vi "Array2HSVColorPic.vi"(0 "Intensity":dbl[][](array[numeric]), 1 "Threshold (max)":dbl, 2 "Threshold (min)":dbl, 3 "Lifetime":dbl[][](array[numeric]), 4 "lifetime_max (s)":dbl=1e-05, 5 "lifetime_min (s)":dbl, 6 "Pic Reference":refnum<vi>, 7 "Auto Scale?":bool) -> (14 "Gray Picture":picture caption="HSV to RGB Picture")   [LabVIEW 2018]
uses:
  <vilib>/picture/picture.llb/Draw True-Color Pixmap.vi
panel:
  in  "hue_min [red]":dbl
  in  "hue_max [blue]":dbl=0.7
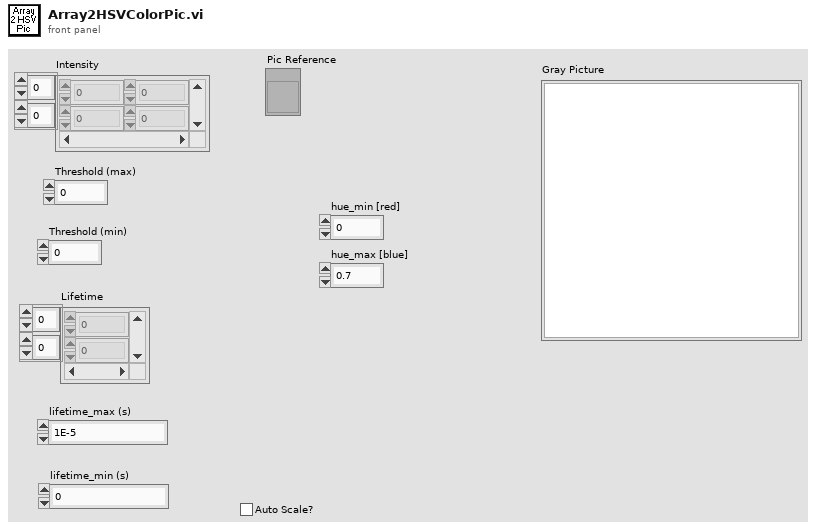
[diagram p1: front panel]
types:
  T1 = typedef "LVBoundsTypeDef.ctl" = cluster{"Width":u32, "Height":u32}
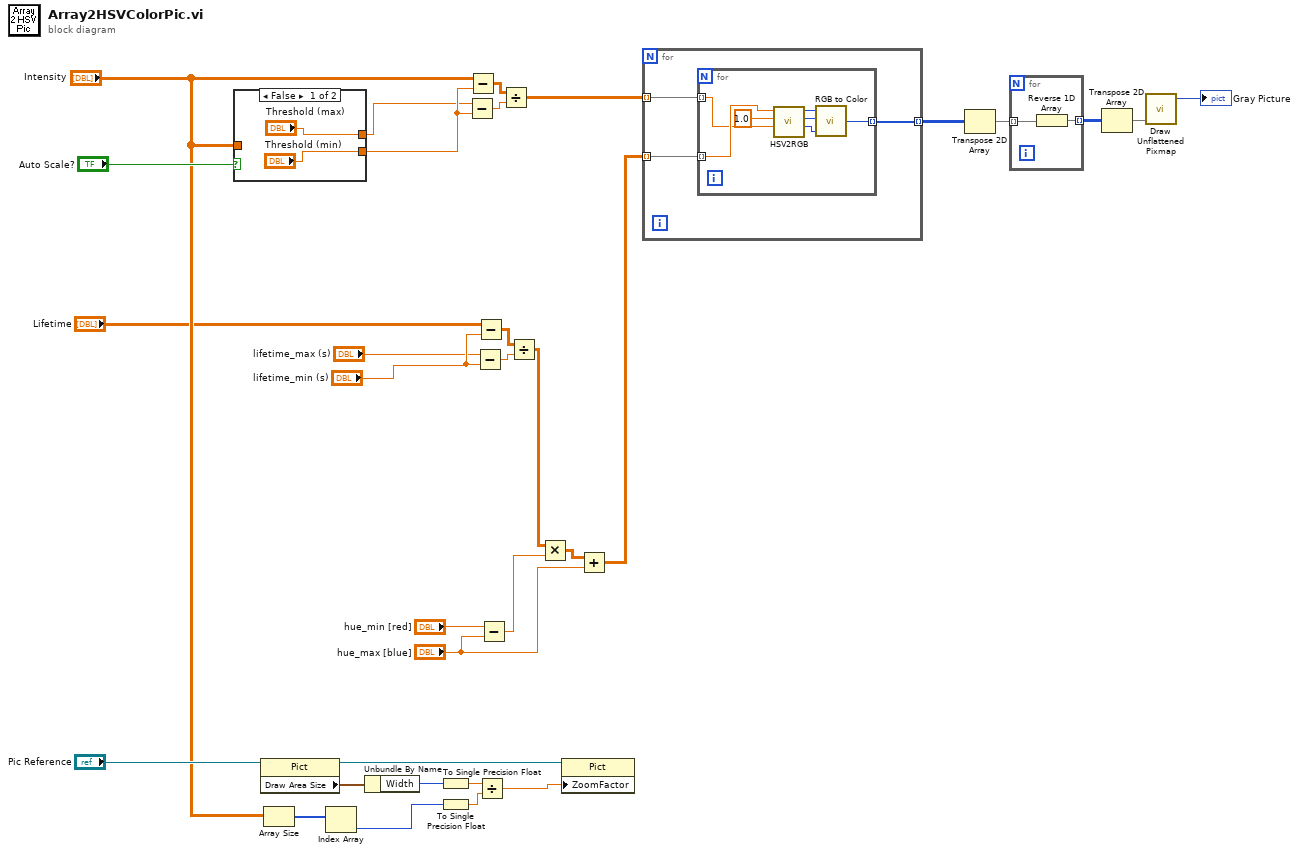
[diagram p0: block diagram]
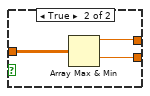
[diagram p2: hidden frame]
diagram:
  n1 = case shown="False" "Auto Scale?" {
    tunnel: "Intensity" -> [_ w37]
    tunnel: ["Threshold (max)" w36] -> w28
    tunnel: ["Threshold (min)" w35] -> w29
    frame False {
    }
    frame True {
      n2 = Array Max & Min(array=w37) -> (max value=w36:dbl, min value=w35:dbl)  [unwired: 2 out]
    }
  }
  n3 = property on="Property Node" class="Pict"(reference="Pic Reference") -> (reference out=w17:refnum<vi>, "Draw Area Size"=w19:T1)  [unwired: 1 in, 1 out]
  n4 = Array Size(array="Intensity") -> (size(s)=w15:i32[])
  n5 = Index Array(array=w15) -> (element=w14:i32)  [unwired: 1 in]
  n6 = Unbundle By Name(w19) -> ("Width"=w23:u32)
  n7 = To Single Precision Float(number=w23) -> (single precision float=w21:sgl)
  n8 = To Single Precision Float(number=w14) -> (single precision float=w22:sgl)
  n9 = Subtract(x=w28, y=w29) -> (x-y=w32:dbl)
  n10 = Subtract(x="Intensity", y=w29) -> (x-y=w31:dbl[][])
  n11 = Subtract(x="lifetime_max (s)", y="lifetime_min (s)") -> (x-y=w12:dbl)
  n12 = Subtract(x="Lifetime", y="lifetime_min (s)") -> (x-y=w13:dbl[][])
  n13 = Divide(x=w21, y=w22) -> (x/y=w18:sgl)
  n14 = Subtract(x="hue_min [red]", y="hue_max [blue]") -> (x-y=w9:dbl)
  n15 = Divide(x=w31, y=w32) -> (x/y=w4:dbl[][])
  n16 = Divide(x=w13, y=w12) -> (x/y=w8:dbl[][])
  n17 = Multiply(x=w8, y=w9) -> (x*y=w1:dbl[][])
  n18 = property on="Property Node" class="Pict"(reference=w17, "ZoomFactor"=w18) -> ()  [unwired: 1 in, 2 out]
  n19 = Add(x=w1, y="hue_max [blue]") -> (x+y=w3:dbl[][])
  n20 = for {
    tunnel: w4 -> [w40] mode=indexing
    tunnel: [w39] -> w2 mode=indexing
    tunnel: w3 -> [w38] mode=indexing
    n21 = for {
      tunnel: w40 -> [w44] mode=indexing
      tunnel: [w47] -> w39 mode=indexing
      tunnel: w38 -> [w45] mode=indexing
      n22 = call "HSV2RGB.vi"("Value"=w44, "Saturation"=1.0, "Hue [0-1)"=w45) -> ("Blue"=w41:u8, "Green"=w42:u8, "Red"=w43:u8)  [unwired: 6 in]
      n23 = call <vilib>:"RGB to Color.vi"("B"=w41, "G"=w42, "R"=w43) -> ("Color"=w47:u32)
    }
  }
  n24 = Transpose 2D Array(2D array=w2) -> (transposed array=w26:u32[][])
  n25 = for {
    tunnel: w26 -> [w49] mode=indexing
    tunnel: [w48] -> w25 mode=indexing
    n26 = Reverse 1D Array(array=w49) -> (reversed array=w48:u32[])
  }
  n27 = Transpose 2D Array(2D array=w25) -> (transposed array=w24:u32[][])
  n28 = call-poly <vilib>:"Draw Unflattened Pixmap.vi"("data (RGB format)"=w24) -> ("new picture"=→"Gray Picture":picture)  [unwired: 8 in]
